vi "Write.vi"(8 "error in":errorcluster, 10 "command":string, 11 "VISA resource name":refnum<visa-resource-name>) -> (0 "error out":errorcluster, 3 "VISA resource name out":refnum<visa-resource-name>)   [LabVIEW 2019, in "Andeen-Hagerling 2700(400 firmware).lvlib"]
doc: "Write a command to the bridge."
uses:
  Andeen-Hagerling 2700(400 firmware).lvlib
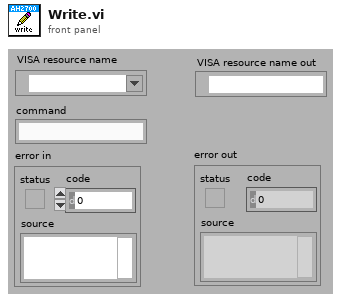
[diagram p1: front panel]
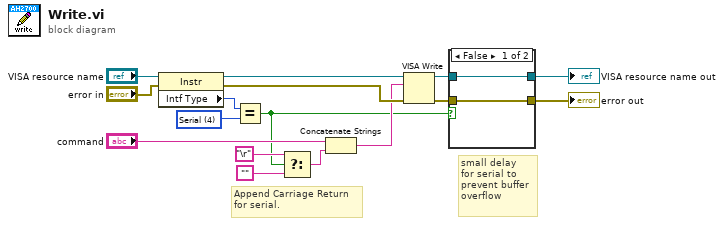
[diagram p0: block diagram]
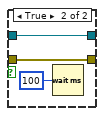
[diagram p2: hidden frame]
diagram:
  w12 = u16 4 items=["GPIB"=1, "VXI"=2, "GPIB-VXI"=3, "Serial"=4, "PXI"=5, "TCPIP"=6, "USB"=7, "FireWire"=9] ("Interface Information:Interface Type")
  # "small delay\nfor serial to \nprevent buffer\noverflow"
  # "Append Carriage Return\nfor serial."
  n1 = property class="Instr"(reference="VISA resource name", error in="error in") -> (reference out=w16:refnum<visa-resource-name>, error out=w15:errorcluster, "Intf Type"=w13:u16)
  n2 = Equal?(x=w13, y=w12) -> (x = y?=w1:bool)
  n3 = Select(t="\r", s=w1, f="") -> (s? t:f=w2:string)
  n4 = Concatenate Strings("command", w2) -> (w5:string)
  n5 = VISA Write(VISA resource name=w16, write buffer=w5, error in (no error)=w15) -> (VISA resource name out=w10:refnum<visa-resource-name>, error out=w8:errorcluster)  [unwired: 1 out]
  n6 = case shown="False" w1 {
    tunnel: w10 -> [w18 w21]
    tunnel: [w18 w21] -> w9
    tunnel: w8 -> [w17 w20]
    tunnel: [w17 w20] -> w7
    frame False {
    }
    frame True {
      n7 = Wait (ms)(milliseconds to wait=u32 100) -> ()  [unwired: 1 out]
    }
  }
  "VISA resource name out" <- w9
  "error out" <- w7
